vi "RecordWave_multi_cards.vi"() -> ()   [LabVIEW 2016]
panel:
  out "About":string
  in  "card #":u32
  in  "card #":u32=1
  out "error out 2":errorcluster
  out "Waveform Graph 2":i32[][](graph)
  out "Rec Error 2":errorcluster
  in  "Stop 2":bool
  out "Device Names":string[](array[string])
  out "Number of Input Devices":i32=2
  out "error out":errorcluster
  out "Rec Error":errorcluster
  in  "Format":cluster{"Rate":i32, "Bits":i32, "Channels":i32}={"Rate"=44100, "Bits"=16, "Channels"=2}
  in  "Buffer":T1={"# buffers"=10, "Buffer size"=50, "unit (ms)"=enum."time (ms)"}
  out "Waveform Graph":i32[][](graph)
  in  "Stop":bool
  # "Record from multiple sound cards"
  # "Soundcard #1"
  # "ONLY for Information\nHas no effect in the code !"
  # "Soundcard #2"
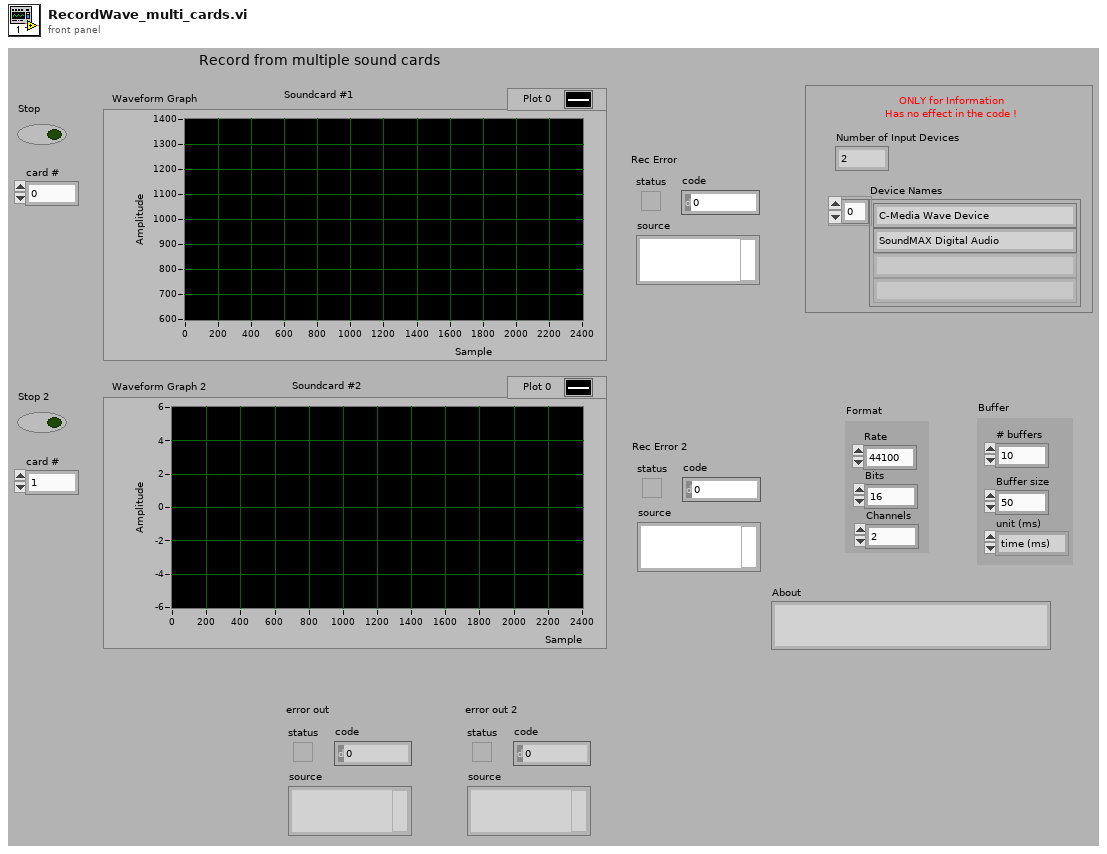
[diagram p1: front panel]
types:
  T1 = cluster{"# buffers":i32, "Buffer size":i32, "unit (ms)":enum16{"time (ms)", "Samples"}}
  T2 = typedef "SoundHandle.ctl" = cluster{"DeviceID":u16, "Samples/buf":u32, "Sampl rate":u32, "Bits/sample":u16, "Channels":u8, "Opened":bool}
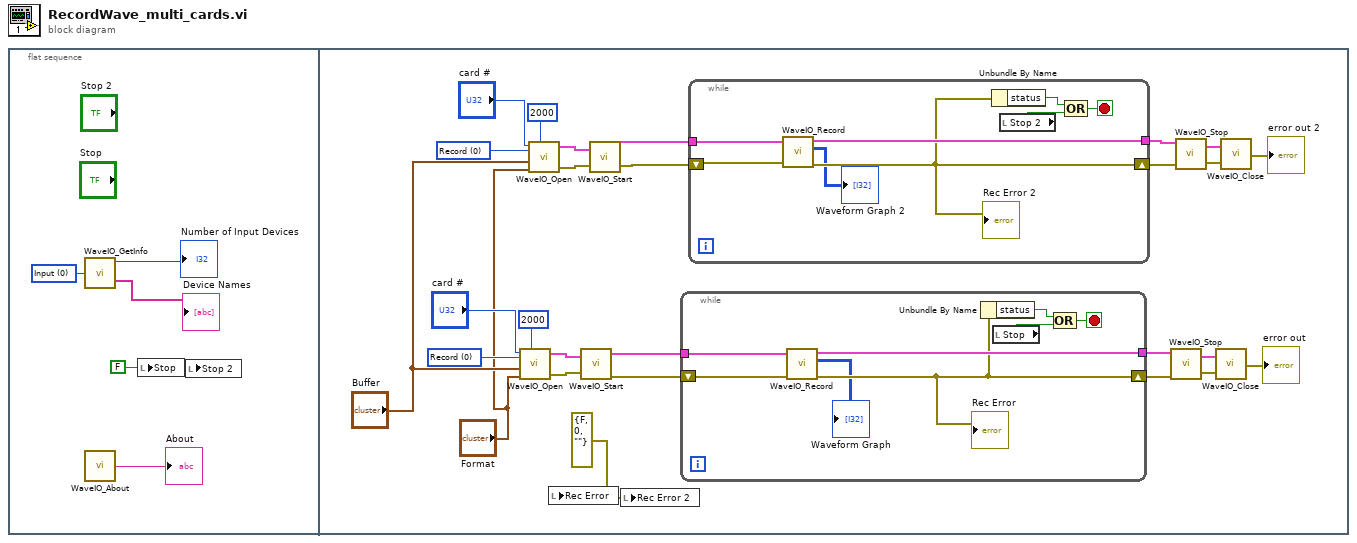
[diagram p0: block diagram]
diagram:
  n1 = flat-sequence {
    frame #0 {
      w3 = u16 0 items=["Input", "Output"] ("Direction (Input)")
      w2 = FALSE ("Stop")
      n2 = call "WaveIO_GetInfo.vi"("Direction (Input)"=w3) -> ("numdev"=→"Number of Input Devices":i32, "Dev Names"=→"Device Names":string[])  [unwired: 2 out]
      n3 = call "WaveIO_About.vi"() -> ("About"=→"About":string)  [unwired: 1 in]
      n4 = local write "Stop"(w2) -> ()
      n5 = local write "Stop 2"(w2) -> ()
    }
    frame #1 {
      w13 = u16 0 items=["Record", "Play"] ("Direction (Record)")
      w6 = errorcluster {"status"=FALSE, "code"=0, "source"=""} ("error in (no error)")
      w24 = u16 0 items=["Record", "Play"] ("Direction (Record)")
      n6 = call "WaveIO_Open.vi"("idev"="card #", "Watchdog timeout (msec) (default=OFF)"=2000, "device type (Record)"=w24, "Buffer Config"="Buffer", "Format (44kHz, 16Bit, stereo)"="Format") -> ("Sound Handle Out"=w27:T2, "error out"=w29:errorcluster)  [unwired: 2 in]
      n7 = call "WaveIO_Open.vi"("idev"="card #", "Watchdog timeout (msec) (default=OFF)"=2000, "device type (Record)"=w13, "Buffer Config"="Buffer", "Format (44kHz, 16Bit, stereo)"="Format") -> ("Sound Handle Out"=w14:T2, "error out"=w10:errorcluster)  [unwired: 2 in]
      n8 = local write "Rec Error"(w6) -> ()
      n9 = call "WaveIO_Start.vi"("error in (no error)"=w29, "Handle"=w27) -> ("error out"=w25:errorcluster, "Handle Out"=w26:T2)
      n10 = call "WaveIO_Start.vi"("error in (no error)"=w10, "Handle"=w14) -> ("error out"=w11:errorcluster, "Handle Out"=w9:T2)
      n11 = local write "Rec Error 2"(w6) -> ()
      n12 = while {
        shift-right: [w44] -> w23
        shift-left: w25 -> [w42]
        tunnel: w26 -> [w41]
        tunnel: [w45] -> w31
        stop <- w48 stop-if-true
        n13 = call "WaveIO_Record.vi"("Handle"=w41, "error in (no error)"=w42) -> ("Handle Out"=w45:T2, "Data"=→"Waveform Graph":i32[][], "error out"=w44:errorcluster)  [unwired: 1 in, 2 out]
        "Rec Error" <- w44
        n14 = Unbundle By Name(w44) -> ("status"=w47:bool)
        n15 = local read "Stop"() -> (w46:bool)
        n16 = Compound Arithmetic op=OR(w47, w46) -> (w48:bool)
      }
      n17 = while {
        shift-right: [w36] -> w16
        shift-left: w11 -> [w33]
        tunnel: w9 -> [w34]
        tunnel: [w37] -> w17
        stop <- w40 stop-if-true
        n18 = call "WaveIO_Record.vi"("Handle"=w34, "error in (no error)"=w33) -> ("Handle Out"=w37:T2, "Data"=→"Waveform Graph 2":i32[][], "error out"=w36:errorcluster)  [unwired: 1 in, 2 out]
        "Rec Error 2" <- w36
        n19 = Unbundle By Name(w36) -> ("status"=w39:bool)
        n20 = local read "Stop 2"() -> (w38:bool)
        n21 = Compound Arithmetic op=OR(w39, w38) -> (w40:bool)
      }
      n22 = call "WaveIO_Stop.vi"("error in (no error)"=w23, "Handle"=w31) -> ("error out"=w28:errorcluster, "Handle Out"=w32:T2)
      n23 = call "WaveIO_Stop.vi"("error in (no error)"=w16, "Handle"=w17) -> ("error out"=w19:errorcluster, "Handle Out"=w20:T2)
      n24 = call "WaveIO_Close.vi"("error in (no error)"=w28, "Handle"=w32) -> ("error out"=→"error out":errorcluster)  [unwired: 1 out]
      n25 = call "WaveIO_Close.vi"("error in (no error)"=w19, "Handle"=w20) -> ("error out"=→"error out 2":errorcluster)  [unwired: 1 out]
    }
  }
